vi "Datasheet Generate SW Calibration File.vi"(8 "error in (no error)":errorcluster, 10 "Destination Directory (Temp)":path, 11 "File Information":T1) -> (0 "error out":errorcluster, 3 "SW Cal File Path":path)   [LabVIEW 2011]
uses:
  TDMS/TDMS File.ctl
  TDMS/TDMS Run.ctl
  TDMS/TDMS Channel (Sxx).ctl
  database/Fields/Field Record.ctl
  database/Fields/Field DataTypes.ctl
  database/Fields/Field NextItem.ctl
  <vilib>/Utility/config.llb/Write Key (String).vi
  <vilib>/Utility/config.llb/Read Key (String).vi
  <vilib>/Utility/config.llb/NI_LVConfig.lvlib
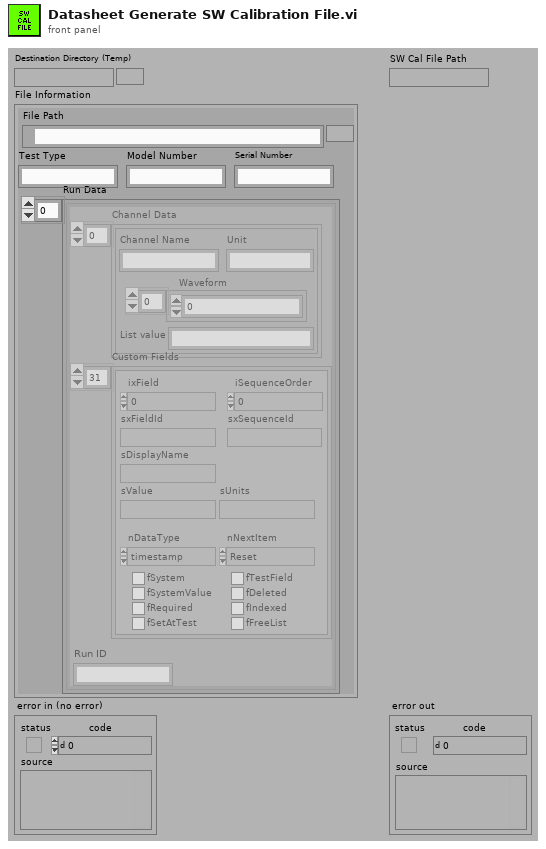
[diagram p1: front panel]
types:
  T1 = typedef "TDMS File.ctl" = cluster{"File Path":path, "Run Data":T2[], "Serial Number":string, "Model Number":string, "Test Type":string}
  T2 = typedef "TDMS Run.ctl" = cluster{"Channel Data":T3[], "Custom Fields":T4[], "Run ID":string}
  T3 = typedef "TDMS Channel (Sxx).ctl" = cluster{"Channel Name":string, "Waveform":dbl[], "Unit":string, "List value":string}
  T4 = typedef "Field Record.ctl" = cluster{"ixField":i32, "iSequenceOrder":i32, "sxFieldId":string, "sxSequenceId":string, "sDisplayName":string, "sValue":string, "sUnits":string, "nDataType":T5, "nNextItem":T6, "fSystem":bool, "fSystemValue":bool, "fRequired":bool, "fSetAtTest":bool, "fTestField":bool, "fDeleted":bool, "fIndexed":bool, "fFreeList":bool}
  T5 = typedef "Field DataTypes.ctl" = enum32{"text", "numeric", "list", "timestamp", "boolean"}
  T6 = typedef "Field NextItem.ctl" = enum32{"Reset", "Retain", "Auto-Increment"}
  T7 = typedef "NI_LVConfig.lvlib/Config Data RefNum.ctl" = refnum<k1>
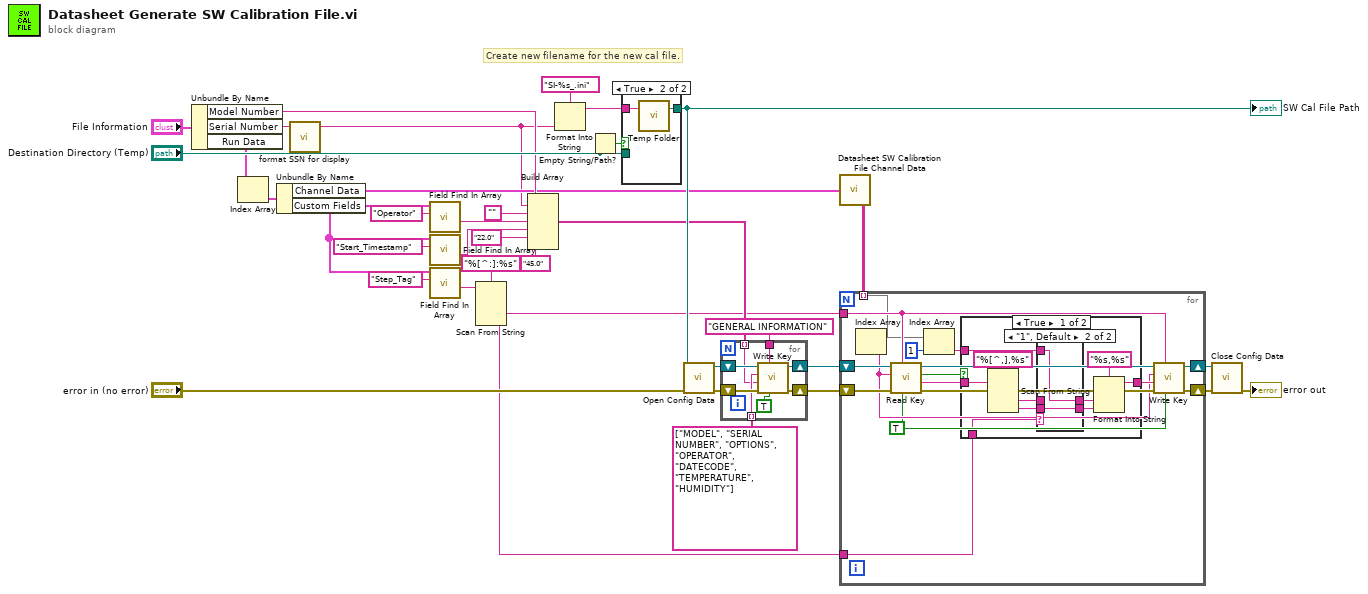
[diagram p0: block diagram]
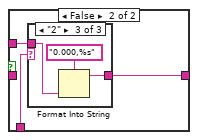
[diagram p3: hidden frame]
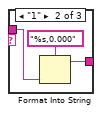
[diagram p5: hidden frame]
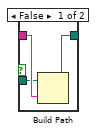
[diagram p6: hidden frame]
diagram:
  # "Create new filename for the new cal file."
  n1 = Unbundle By Name("File Information") -> ("Model Number"=w19:string, "Serial Number"=w36:string, "Run Data"=w11:T2[])
  n2 = Index Array(array=w11) -> (element=w33:T2)  [unwired: 1 in]
  n3 = Unbundle By Name(w33) -> ("Channel Data"=w10:T3[], "Custom Fields"=w8:T4[])
  n4 = call "format SSN for display.vi"("string"=w36) -> ("s? t:f"=w1:string)  [unwired: 4 out]
  n5 = call "Field Find In Array.vi"("FieldID or Display Name(\"\")"="Operator" ("format string"), "Field Array"=w8) -> ("sValue"=w17:string)  [unwired: 1 in, 8 out]
  n6 = call "Field Find In Array.vi"("FieldID or Display Name(\"\")"="Start_Timestamp" ("format string"), "Field Array"=w8) -> ("sValue"=w16:string)  [unwired: 1 in, 8 out]
  n7 = call "Field Find In Array.vi"("FieldID or Display Name(\"\")"="Step_Tag" ("format string"), "Field Array"=w8) -> ("sValue"=w7:string)  [unwired: 1 in, 8 out]
  n8 = Scan From String(format string="%[^:]:%s", input string=w7) -> (output 1=w3:string, output 2=w2:string)  [unwired: 4 in, 3 out]
  n9 = Build Array(w19, w1, "", w17, w16, "22.0" ("format string"), "45.0" ("format string")) -> (w12:string[])
  n10 = Format Into String(format string="SI-%s_.ini", w1) -> (resulting string=w31:string)  [unwired: 2 in, 1 out]
  n11 = Empty String/Path?(string/path="Destination Directory (Temp)") -> (empty?=w30:bool)
  n12 = case shown="True" w30 {
    tunnel: [w40 w42] -> w21
    tunnel: w31 -> [w39 w41]
    tunnel: "Destination Directory (Temp)" -> [w38 _]
    frame False {
      n13 = Build Path(base path=w38, name or relative path=w39) -> (appended path=w40:path)
    }
    frame True {
      n14 = call "Temp Folder.vi"("Relative Path (\"\")"=w41) -> ("Temp Folder"=w42:path)  [unwired: 2 in]
    }
  }
  "SW Cal File Path" <- w21
  n15 = call <vilib>:"Open Config Data.vi"("error in (no error)"="error in (no error)", "configuration file path"=w21) -> ("error out"=w28:errorcluster, "refnum"=w26:T7)  [unwired: 7 in, 1 out]
  n16 = for {
    tunnel: "GENERAL INFORMATION" ("format string") -> [w46]
    tunnel: string[] ["MODEL", "SERIAL NUMBER", "OPTIONS", "OPERATOR", "DATECODE", "TEMPERATURE", "HUMIDITY"] -> [w45] mode=indexing
    shift-right: [w48] -> w25
    shift-left: w28 -> [w50]
    shift-right: [w47] -> w22
    shift-left: w26 -> [w49]
    tunnel: w12 -> [w44] mode=indexing
    n17 = call-poly <vilib>:"Write Key.vi"("write raw string? (F)"=TRUE, "section"=w46, "error in (no error)"=w50, "value"=w44, "key"=w45, "refnum"=w49) -> ("error out"=w48:errorcluster, "refnum out"=w47:T7)  [unwired: 3 in, 1 out]
  }
  n18 = call "Datasheet SW Calibration File Channel Data.vi"("Channel Data"=w10) -> ("Formatted Channel Values"=w4:string[][])
  n19 = for {
    shift-right: [w66] -> w24
    shift-left: w25 -> [w63]
    shift-right: [w65] -> w23
    shift-left: w22 -> [w64]
    tunnel: w4 -> [w54] mode=indexing
    tunnel: w3 -> [w60]
    tunnel: w2 -> [w51]
    w52 = TRUE ("read raw string? (F)")
    n20 = Index Array(array=w54) -> (element=w53:string)  [unwired: 1 in]
    n21 = call-poly <vilib>:"Read Key.vi"("read raw string? (F)"=w52, "section"=w60, "error in (no error)"=w63, "key"=w53, "refnum"=w64) -> ("error out"=w62:errorcluster, "value"=w56:string, "found?"=w58:bool, "refnum out"=w61:T7)  [unwired: 3 in]
    n22 = Index Array(array=w54, index=1) -> (element=w57:string)
    n23 = case shown="True" w58 {
      tunnel: w57 -> [w76 w83]
      tunnel: w56 -> [w67 _]
      tunnel: [w72 w81] -> w55
      tunnel: w51 -> [w74 w82]
      frame True {
        n24 = Scan From String(format string="%[^,],%s", input string=w67) -> (output 1=w68:string, output 2=w73:string)  [unwired: 4 in, 3 out]
        n25 = case shown="\"1\", Default" w74 {
          tunnel: w76 -> [w78 w80]
          tunnel: w68 -> [w77 _]
          tunnel: w73 -> [_ w79]
          tunnel: [w77 w80] -> w71
          tunnel: [w78 w79] -> w69
          frame "2" {
          }
          frame "1", Default {
          }
        }
        n26 = Format Into String(format string="%s,%s", w71, w69) -> (resulting string=w72:string)  [unwired: 2 in, 1 out]
      }
      frame False {
        n27 = case shown="\"2\"" w82 {
          tunnel: w83 -> [w84 w85 w88]
          tunnel: [w84 w86 w89] -> w81
          frame Default {
          }
          frame "1" {
            n28 = Format Into String(format string="%s,0.000", w85) -> (resulting string=w86:string)  [unwired: 2 in, 1 out]
          }
          frame "2" {
            n29 = Format Into String(format string="0.000,%s", w88) -> (resulting string=w89:string)  [unwired: 2 in, 1 out]
          }
        }
      }
    }
    n30 = call-poly <vilib>:"Write Key.vi"("write raw string? (F)"=w52, "section"=w60, "error in (no error)"=w62, "value"=w55, "key"=w53, "refnum"=w61) -> ("error out"=w66:errorcluster, "refnum out"=w65:T7)  [unwired: 3 in, 1 out]
  }
  n31 = call <vilib>:"Close Config Data.vi"("error in (no error)"=w24, "refnum"=w23) -> ("error out"=→"error out":errorcluster)  [unwired: 8 in, 1 out]
